vi "PathPlanner_Trajectory25_GenerateStates_Pass2.vi"(9 "RobotConfig":T1 {"moduleLocations"."Y" format="%14.3f"; "moduleLocations"."X" format="%14.3f"; "ModuleConfig"."driveMotor"."Jr_KgM2" format="%13.5p"; "ModuleConfig"."driveMotor"."L_H" format="%13.5p"; "ModuleConfig"."driveMotor"."Kt_NMPerAmp" format="%13.5p"; "ModuleConfig"."driveMotor"."KvINV_RadPerSecPerVolt" format="%13.5p"; "ModuleConfig"."driveMotor"."R_Ohms" format="%13.5p"; "ModuleConfig"."driveMotor"."FreeSpeed_RadPerSec" format="%13.5p"; "ModuleConfig"."driveMotor"."FreeCurrent_Amps" format="%13.5p"; "ModuleConfig"."driveMotor"."StallCurrent_Amps" format="%13.5p"; "ModuleConfig"."driveMotor"."StallTorque_NM" format="%13.5p"; "ModuleConfig"."driveMotor"."nominalVoltage_Volts" format="%13.5p"}, 11 "in PathPlannerStates":T5[](array[typedef]) {"ModuleStates"."SWERVE_DRIVE_MODULE_STATE"."Angle"."SIN" format="%13.4f"; "ModuleStates"."SWERVE_DRIVE_MODULE_STATE"."Angle"."COS" format="%13.4f"; "ModuleStates"."SWERVE_DRIVE_MODULE_STATE"."Angle"."VALUE" format="%13.4f"; "ModuleStates"."FieldAngle"."SIN" format="%13.4f"; "ModuleStates"."FieldAngle"."COS" format="%13.4f"; "ModuleStates"."FieldAngle"."VALUE" format="%13.4f"; "ModuleStates"."FieldPos"."Y" format="%14.3f"; "ModuleStates"."FieldPos"."X" format="%14.3f"; "DeltaRot"."SIN" format="%13.4f"; "DeltaRot"."COS" format="%13.4f"; "DeltaRot"."VALUE" format="%13.4f"; "pose"."ROTATION"."SIN" format="%13.4f"; "pose"."ROTATION"."COS" format="%13.4f"; "pose"."ROTATION"."VALUE" format="%13.4f"; "pose"."TRANSLATION"."Y" format="%14.3f"; "pose"."TRANSLATION"."X" format="%14.3f"; "FieldSpeeds"."vOmega" format="%10.3f"; "FieldSpeeds"."vY" format="%10.3f"; "FieldSpeeds"."vX" format="%10.3f"; "Heading"."SIN" format="%13.4f"; "Heading"."COS" format="%13.4f"; "Heading"."VALUE" format="%13.4f"}) -> (3 "out PathPlannerStates":T5[](array[typedef]) {"ModuleStates"."SWERVE_DRIVE_MODULE_STATE"."Angle"."SIN" format="%13.4f"; "ModuleStates"."SWERVE_DRIVE_MODULE_STATE"."Angle"."COS" format="%13.4f"; "ModuleStates"."SWERVE_DRIVE_MODULE_STATE"."Angle"."VALUE" format="%13.4f"; "ModuleStates"."FieldAngle"."SIN" format="%13.4f"; "ModuleStates"."FieldAngle"."COS" format="%13.4f"; "ModuleStates"."FieldAngle"."VALUE" format="%13.4f"; "ModuleStates"."FieldPos"."Y" format="%14.3f"; "ModuleStates"."FieldPos"."X" format="%14.3f"; "DeltaRot"."SIN" format="%13.4f"; "DeltaRot"."COS" format="%13.4f"; "DeltaRot"."VALUE" format="%13.4f"; "pose"."ROTATION"."SIN" format="%13.4f"; "pose"."ROTATION"."COS" format="%13.4f"; "pose"."ROTATION"."VALUE" format="%13.4f"; "pose"."TRANSLATION"."Y" format="%14.3f"; "pose"."TRANSLATION"."X" format="%14.3f"; "FieldSpeeds"."vOmega" format="%10.3f"; "FieldSpeeds"."vY" format="%10.3f"; "FieldSpeeds"."vX" format="%10.3f"; "Heading"."SIN" format="%13.4f"; "Heading"."COS" format="%13.4f"; "Heading"."VALUE" format="%13.4f"})   [LabVIEW 2019, in "PathPlanner24.lvlib"]
doc: "Internal routine to help create a trajectory from a path."
uses:
  <vilib>/Rock Robotics/WPI/ThirdParty/JAS_Junk/TrajLib/TypeDef/TRANSLATION2D.ctl
  <vilib>/Rock Robotics/WPI/ThirdParty/JAS_Junk/TrajLib/TypeDef/ROTATION2D.ctl
  TypeDef/PathPlannerPathConstraints.ctl
  PathPlanner24.lvlib
  <vilib>/Rock Robotics/WPI/ThirdParty/JAS_Junk/TrajLib/Trajectory_Library.lvlib
  <vilib>/Rock Robotics/WPI/ThirdParty/JAS_Junk/TrajLib/TypeDef/CHASSIS_SPEEDS.ctl
  <vilib>/Rock Robotics/WPI/ThirdParty/JAS_Junk/TrajLib/TypeDef/POSE2D.ctl
  <vilib>/Rock Robotics/WPI/ThirdParty/JAS_Junk/TrajLib/TypeDef/SWERVE_DRIVE_MODULE_STATE.ctl
  TypeDef/PathPlannerSwerveModTrajState.ctl
  TypeDef/PathPlannerDriveFeedFwds.ctl
  TypeDef/PathPlannerTrajectoryState25.ctl
  <vilib>/Rock Robotics/WPI/ThirdParty/JAS_Junk/TrajLib/TypeDef/DCMOTOR.CTL
  TypeDef/PathPlannerModuleConfig.ctl
  TypeDef/PathPlannerRobotConfig.ctl
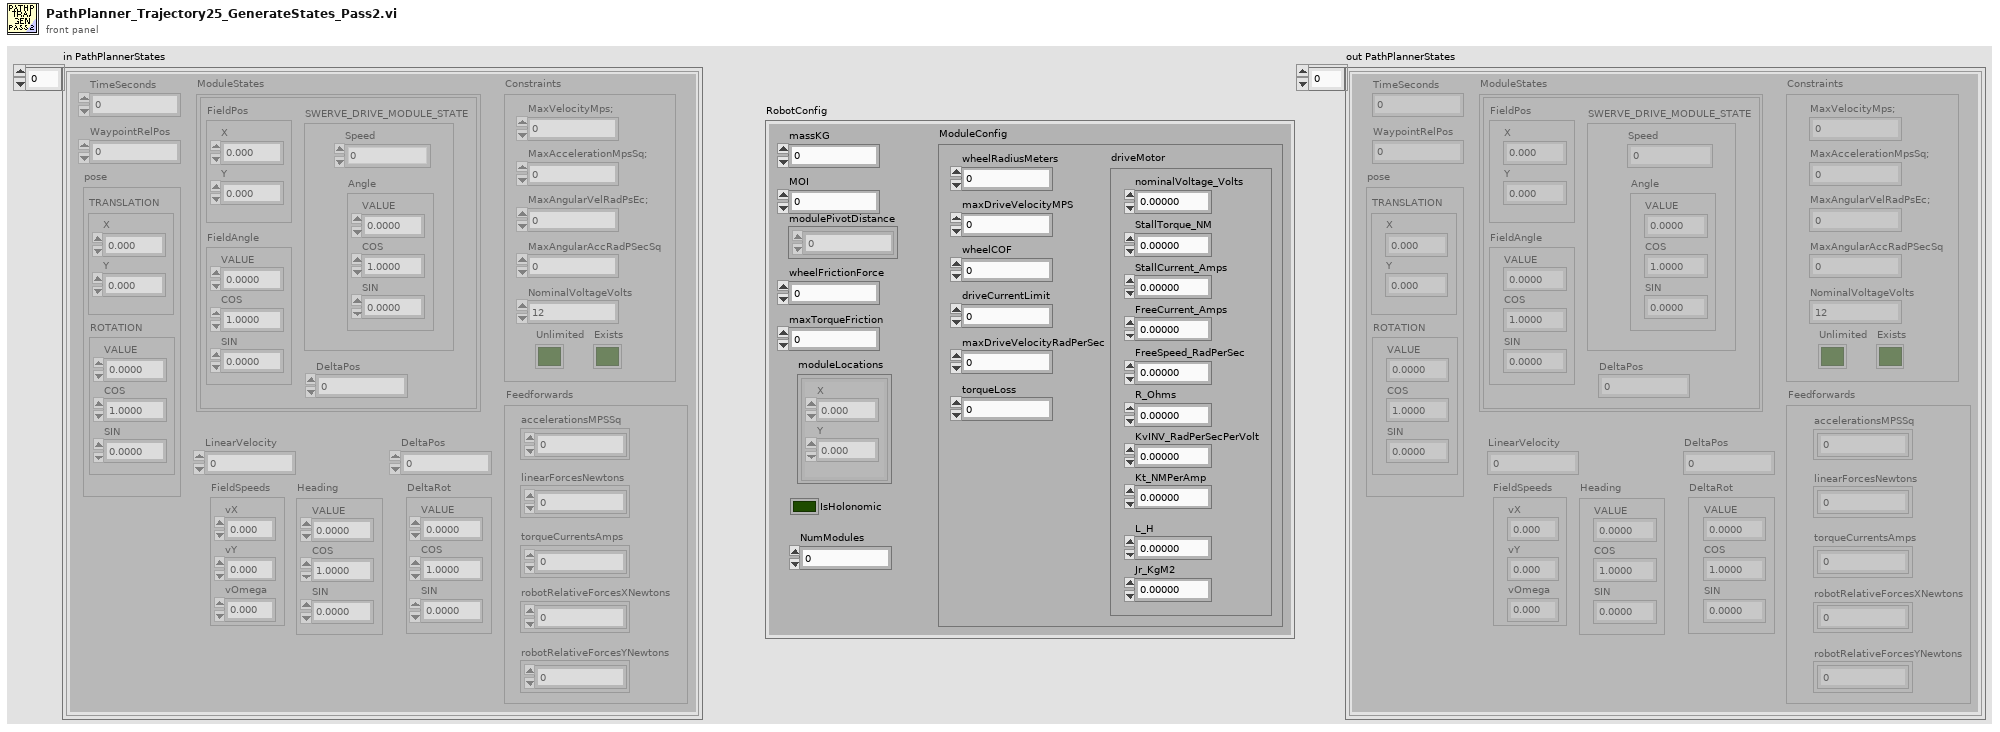
[diagram p1: front panel]
types:
  T1 = typedef "PathPlanner24.lvlib/PathPlannerRobotConfig.ctl" = cluster{"massKG":dbl, "MOI":dbl, "modulePivotDistance":dbl[], "wheelFrictionForce":dbl, "maxTorqueFriction":dbl, "ModuleConfig":T2, "moduleLocations":T4[], "IsHolonomic":bool, "NumModules":i32}
  T2 = typedef "PathPlanner24.lvlib/PathPlannerModuleConfig.ctl" = cluster{"wheelRadiusMeters":dbl, "maxDriveVelocityMPS":dbl, "wheelCOF":dbl, "driveCurrentLimit":dbl, "maxDriveVelocityRadPerSec":dbl, "torqueLoss":dbl, "driveMotor":T3}
  T3 = typedef "Trajectory_Library.lvlib/DCMOTOR.CTL" = cluster{"nominalVoltage_Volts":dbl, "StallTorque_NM":dbl, "StallCurrent_Amps":dbl, "FreeCurrent_Amps":dbl, "FreeSpeed_RadPerSec":dbl, "R_Ohms":dbl, "KvINV_RadPerSecPerVolt":dbl, "Kt_NMPerAmp":dbl, "L_H":dbl, "Jr_KgM2":dbl}
  T4 = typedef "Trajectory_Library.lvlib/TRANSLATION2D.ctl" = cluster{"X":dbl, "Y":dbl}
  T5 = typedef "PathPlanner24.lvlib/PathPlannerTrajectoryState25.ctl" = cluster{"TimeSeconds":dbl, "LinearVelocity":dbl, "Heading":T6, "Constraints":T7, "DeltaPos":dbl, "FieldSpeeds":T8, "pose":T9, "DeltaRot":T6, "ModuleStates":T10[], "WaypointRelPos":dbl, "Feedforwards":T12}
  T6 = typedef "Trajectory_Library.lvlib/ROTATION2D.ctl" = cluster{"VALUE":dbl, "COS":dbl, "SIN":dbl}
  T7 = typedef "PathPlanner24.lvlib/PathPlannerPathConstraints.ctl" = cluster{"MaxVelocityMps;":dbl, "MaxAccelerationMpsSq;":dbl, "MaxAngularVelRadPsEc;":dbl, "MaxAngularAccRadPSecSq":dbl, "Exists":bool, "Unlimited":bool, "NominalVoltageVolts":dbl}
  T8 = typedef "Trajectory_Library.lvlib/CHASSIS_SPEEDS.ctl" = cluster{"vX":dbl, "vY":dbl, "vOmega":dbl}
  T9 = typedef "Trajectory_Library.lvlib/POSE2D.ctl" = cluster{"TRANSLATION":T4, "ROTATION":T6}
  T10 = typedef "PathPlanner24.lvlib/PathPlannerSwerveModTrajState.ctl" = cluster{"FieldPos":T4, "FieldAngle":T6, "DeltaPos":dbl, "SWERVE_DRIVE_MODULE_STATE":T11}
  T11 = typedef "Trajectory_Library.lvlib/SWERVE_DRIVE_MODULE_STATE.ctl" = cluster{"Speed":dbl, "Angle":T6}
  T12 = typedef "PathPlanner24.lvlib/PathPlannerDriveFeedFwds.ctl" = cluster{"accelerationsMPSSq":dbl[], "linearForcesNewtons":dbl[], "torqueCurrentsAmps":dbl[], "robotRelativeForcesXNewtons":dbl[], "robotRelativeForcesYNewtons":dbl[]}
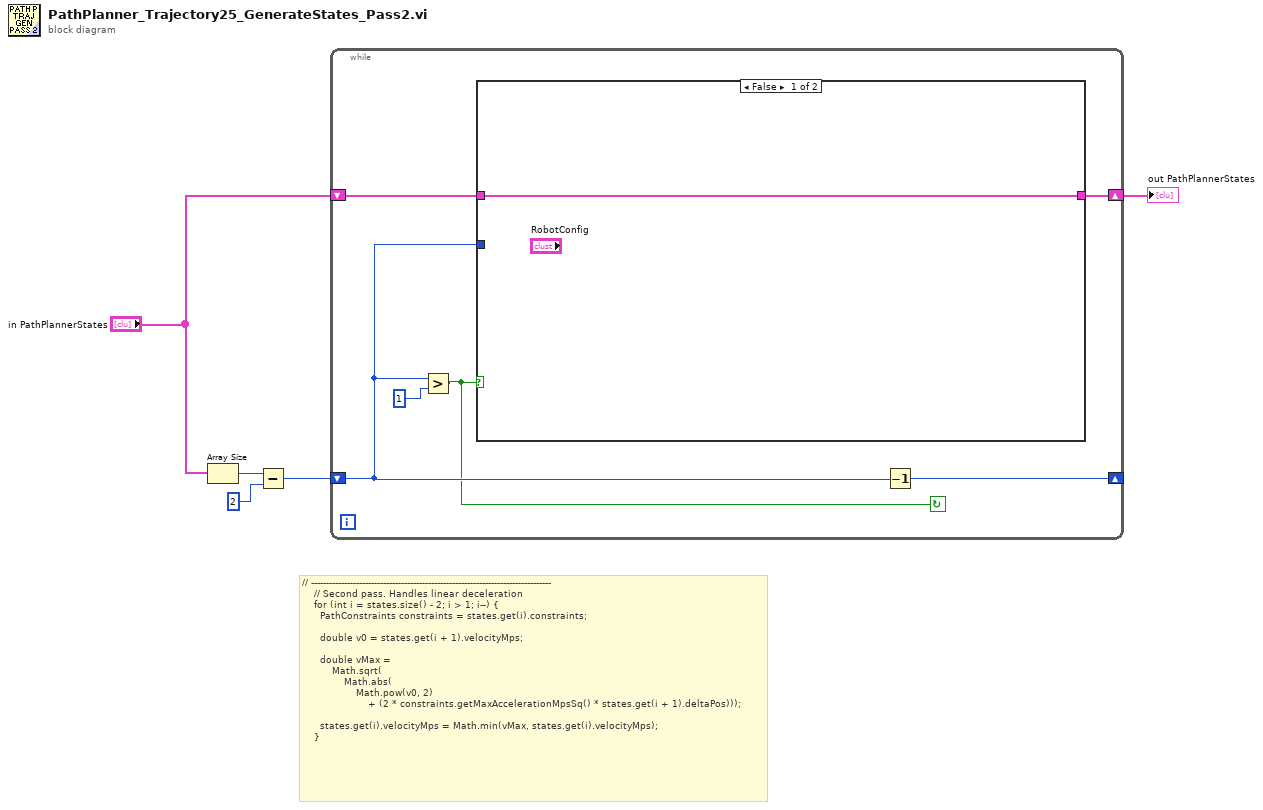
[diagram p0: block diagram]
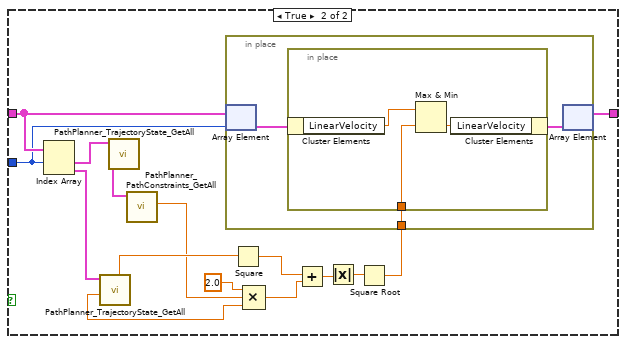
[diagram p2: hidden frame]
diagram:
  # "// --------------------------------------------------------------------------------\n    // Second pass. Handles linear deceleration\n    for (int i = states.size() - 2; i > 1; i--) {\n      PathConstraints constraints = states.get(i).constraints;\n\n      double v0 = states.get(i + 1).velocityMps;\n\n      double vMax =\n          Math.sqrt(\n              Math.abs(\n                  Math.pow(v0, 2)\n                      + (2 * constraints.getMaxAccelerationMpsSq() * states.get(i + 1).deltaPos)));\n\n      states.get(i).velocityMps = Math.min(vMax, states.get(i).velocityMps);\n    }"
  n1 = Array Size(array="in PathPlannerStates") -> (size(s)=w5:i32)
  n2 = Subtract(x=w5, y=2) -> (x-y=w3:i32)
  n3 = while {
    shift-right: [w11] -> _
    shift-left: w3 -> [w8]
    shift-right: [w9] -> w1
    shift-left: "in PathPlannerStates" -> [w10]
    stop <- w6 continue-if-true
    n4 = Greater?(x=w8, y=1) -> (0:w6:bool)
    n5 = case shown="False" w6 {
      tunnel: w10 -> [w12 w25]
      tunnel: w8 -> [_ w24]
      tunnel: [w12 w23] -> w9
      frame False {
      }
      frame True {
        n6 = Index Array(array=w25, index #1=w24) -> (element #1=w27:T5, element #2=w26:T5)  [unwired: 1 in]
        n7 = call "PathPlanner_TrajectoryState_GetAll.vi"("PathPlannerState"=w26) -> ("VelocityMPS"=w22:dbl, "DeltaPos"=w18:dbl)  [unwired: 1 in, 8 out]
        n8 = call "PathPlanner_TrajectoryState_GetAll.vi"("PathPlannerState"=w27) -> ("PathPlannerConstraints"=w20:T7)  [unwired: 1 in, 9 out]
        n9 = call "PathPlanner_PathConstraints_GetAll.vi"("PathPlannerConstraints"=w20) -> ("MaxAccelerationMpsSq;"=w19:dbl)  [unwired: 6 in, 4 out]
        n10 = Square(x=w22) -> (x^2=w16:dbl)
        n11 = Compound Arithmetic op=MULTIPLY(2.0 ("x"), w19, w18) -> (w17:dbl)
        n12 = Add(x=w16, y=w17) -> (x+y=w15:dbl)
        n13 = Absolute Value(x=w15) -> (abs(x)=w14:dbl)
        n14 = Square Root(x=w14) -> (sqrt(x)=w13:dbl)
        n15 = in-place {
          in-place-border: w13 -> [w28]
          n16 = in-place-array #1(w25, w24) -> (w30:T5)
          n17 = in-place {
            in-place-border: w28 -> [w31]
            n18 = in-place-cluster #2(w30) -> ("LinearVelocity"=w32:dbl)
            n19 = Max & Min(x=w32, y=w31) -> (min(x,y)=w33:dbl)  [unwired: 1 out]
            n20 = in-place-cluster #2("LinearVelocity"=w33) -> (w29:T5)
          }
          n21 = in-place-array #1(w29) -> (w23:T5[])  [unwired: 1 out]
        }
      }
    }
    n22 = Decrement(x=w8) -> (x-1=w11:i32)
  }
  "out PathPlannerStates" <- w1
